vi "json_parse_string.vi"(8 "error in (no error)":errorcluster, 11 "data":string) -> (0 "error out":errorcluster, 1 "raw_string":string, 2 "value":variant, 3 "remaining data":string)   [LabVIEW 2017]
uses:
  <vilib>/regexp/Match Regular Expression.xnode
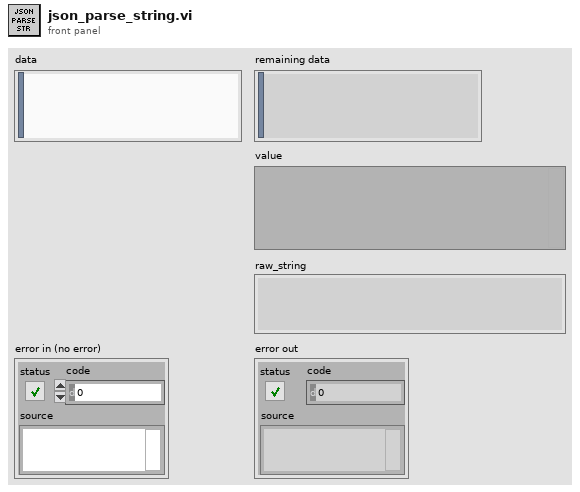
[diagram p1: front panel]
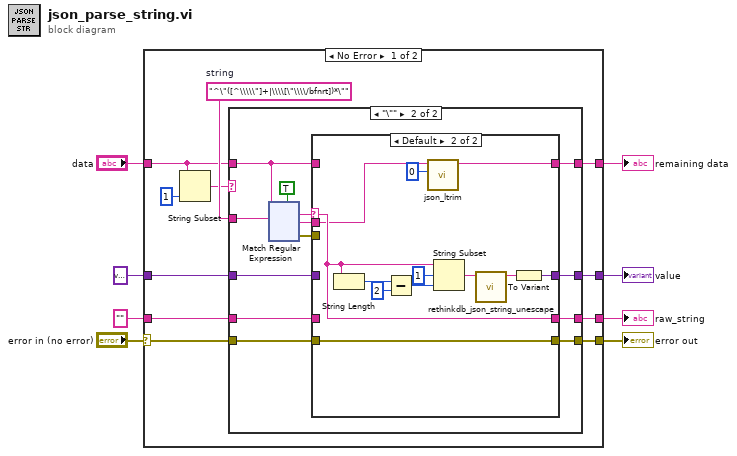
[diagram p0: block diagram]
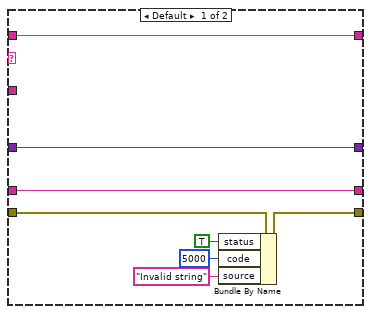
[diagram p2: hidden frame]
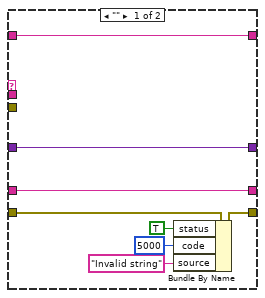
[diagram p3: hidden frame]
diagram:
  n1 = case shown="No Error" "error in (no error)" {
    selector: "error in (no error)" -> [w15 w178]
    tunnel: [w18 w176] -> w8
    tunnel: [w17 w177] -> w7
    tunnel: [w16 w178] -> w6
    tunnel: [w14 w175] -> w4
    tunnel: "data" -> [w13 w176]
    tunnel: variant -> [w10 w177]
    tunnel: "" -> [w9 w175]
    frame No Error {
      w19 = "^\"([^\\\\\"]+|\\\\[\"\\\\/bfnrt])*\""  # string
      n2 = String Subset(string=w13, length (rest)=1 ("length (rest)")) -> (substring=w11:string)  [unwired: 1 in]
      n3 = case shown="\"\\\"\"" w11 {
        tunnel: [w27 w34] -> w17
        tunnel: w10 -> [w27 w35]
        tunnel: [w26 w36] -> w18
        tunnel: w13 -> [w26 w29]
        tunnel: w19 -> [_ w39]
        tunnel: [w21 w33] -> w16
        tunnel: w15 -> [w22 w32]
        tunnel: [w20 w31] -> w14
        tunnel: w9 -> [w20 w28]
        frame Default {
          n4 = Bundle By Name(cluster=w22, "status"=TRUE, "code"=5000, "source"="Invalid string") -> (w21:errorcluster)
        }
        frame "\"" {
          n5 = xnode "Match Regular Expression"("input string"=w29, "regular expression"=w39, "multiline? (F)"=TRUE) -> ("whole match"=w37:string, "after match"=w38:string, "error out"=w30:errorcluster)  [unwired: 3 in, 2 out]
          n6 = case shown="Default" w37 {
            selector: w37 -> [_ w52]
            tunnel: w38 -> [_ w50]
            tunnel: [w48 w49] -> w36
            tunnel: w29 -> [w48 _]
            tunnel: w35 -> [w47 _]
            tunnel: [w47 w58] -> w34
            tunnel: [w45 w53] -> w33
            tunnel: w32 -> [w46 w53]
            tunnel: [w41 w52] -> w31
            tunnel: w30 -> [_ _]
            tunnel: w28 -> [w41 _]
            frame "" {
              n7 = Bundle By Name(cluster=w46, "status"=TRUE, "code"=5000, "source"="Invalid string") -> (w45:errorcluster)
            }
            frame Default {
              n8 = String Length(string=w52) -> (length=w56:i32)
              n9 = Subtract(x=w56, y=2) -> (x-y=w54:i32)
              n10 = call "json_ltrim.vi"("offset (0)"=0, "data"=w50) -> ("left trim whitespace"=w49:string)  [unwired: 9 in]
              n11 = String Subset(string=w52, offset (0)=1, length (rest)=w54) -> (substring=w60:string)
              n12 = call "rethinkdb_json_string_unescape.vi"("escaped string"=w60) -> ("string out"=w59:string)  [unwired: 9 in, 1 out]
              n13 = To Variant(anything=w59) -> (Variant=w58:variant)
            }
          }
        }
      }
    }
    frame Error {
    }
  }
  "remaining data" <- w8
  "value" <- w7
  "error out" <- w6
  "raw_string" <- w4
